vi "MM9.compile header.vi"(0 "i ref in":refnum<vi>, 5 "error in (no error)":errorcluster) -> (14 "i ref out":refnum<vi>, 16 "my header":string, 19 "error out":errorcluster)   [LabVIEW 2014, in "MM9.lvlib"]
doc: "This method compiles the user (Stefan et al.) defined header, that is used in all data files."
uses:
  MM9.lvlib
panel:
  # "This is just for test purposes"
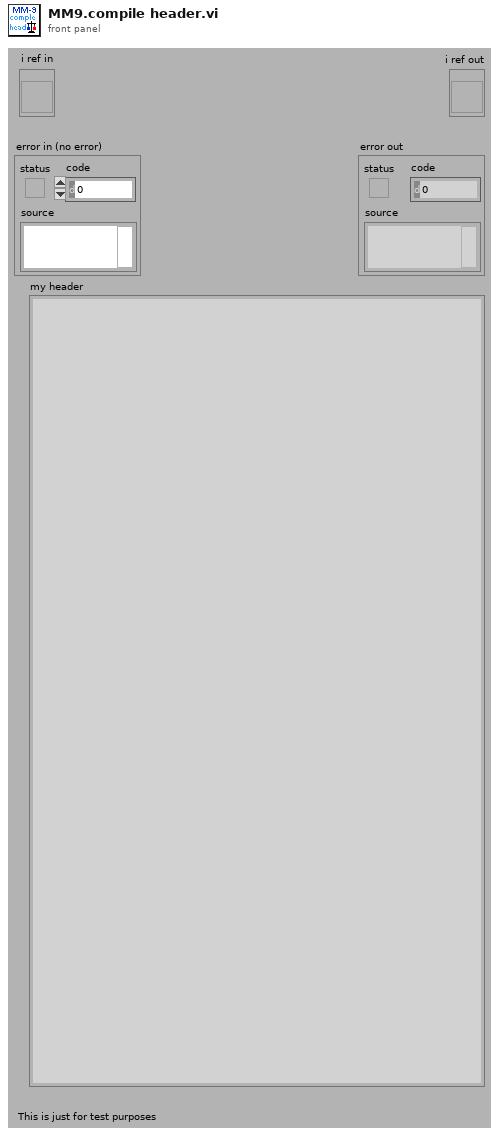
[diagram p1: front panel]
types:
  T1 = typedef "MM9.lvlib/MM9.i attribute.ctl" = cluster{"UsedObjs":string[], "ActScanStep":i32[], "AbortRequest":bool, "StopRequest":bool, "# cycles":i32, "Connected":bool, "MMStatus":T2, "# data":i32, "DIMServices":cluster{"MM6StatusString":string, "MM6StatusID":i32, "discArchiver":string, "discArchiverID":i32, "eventBuilder":string, "eventBuilderID":i32, "GUIIDString":string, "GUIIDStringID":i32}, "dataFile":string, "PGRunning":T3, "ConfigData":T4, "ExtraDataSets":T19}
  T2 = typedef "MM9.lvlib/MM9.status.ctl" = enum16{"loaded", "load_error", "config", "config_error", "init", "init_error", "data_reset", "data_reset_error", "running", "start_error", "run_error", "abort_requested", "aborted", "stop_requested", "stopped", "stop_error", "Connected", "NOTConnected"}
  T3 = typedef "PPG_ABC.lvlib/PPG_ABC.PG_Running.ctl" = i32
  T4 = typedef "LEBITDefs9.lvlib/LEBITDefs.ConfigData.ctl" = cluster{"GenConfig":T5, "Configs":T7[]}
  T5 = typedef "LEBITDefs9.lvlib/LEBITDefs.GenConfig.ctl" = cluster{"Mode":i32, "Logs":T6[]}
  T6 = typedef "LEBITDefs9.lvlib/LEBITDefs.Log.ctl" = cluster{"Name":string, "FctName":string, "Special":string}
  T7 = typedef "LEBITDefs9.lvlib/LEBITDefs.OneConfig.ctl" = cluster{"MCA":T8, "Timing":T9, "Scans":T12[], "FreqDevs":T13[], "CleanDev":T14, "NrCycles":i32, "Specials":T16[], "Delays":T17[], "DAC":T18}
  T8 = typedef "LEBITDefs9.lvlib/LEBITDefs.MCA.ctl" = cluster{"Name":string, "Address":string, "NrChannels":i32, "Gate":i32, "NrPipse":i32, "AcqDelay":i32}
  T9 = typedef "LEBITDefs9.lvlib/LEBITDefs.Timing.ctl" = cluster{"TimeTables":cluster{"TimeTable":T10}[], "Memories":T11[], "ScanX":string, "ScanY":string}
  T10 = typedef "LEBITDefs9.lvlib/LEBITDefs.Timetable.ctl" = dbl[]
  T11 = typedef "LEBITDefs9.lvlib/LEBITDefs.Memory.ctl" = cluster{"Device":string, "ExtTrig":bool, "TT2Use":i32, "PatternTable":string[]}
  T12 = typedef "LEBITDefs9.lvlib/LEBITDefs.ScanDev.ctl" = cluster{"Name":string, "FctName":string, "Values":dbl[], "NrScanVals":i32, "Special":string}
  T13 = typedef "LEBITDefs9.lvlib/LEBITDefs.FreqDev.ctl" = cluster{"Name":string, "Amp":dbl, "CenterFreq":dbl, "Time":dbl}
  T14 = typedef "LEBITDefs9.lvlib/LEBITDefs.CleanDev.ctl" = cluster{"Name":string, "CleanData":T15[]}
  T15 = typedef "LEBITDefs9.lvlib/LEBITDefs.CleanDataType.ctl" = cluster{"Amp":dbl, "Center":dbl, "Plus":dbl, "Minus":dbl, "Time":dbl}
  T16 = typedef "LEBITDefs9.lvlib/LEBITDefs.Special.ctl" = cluster{"Name":string, "FctName":string, "VerySpecial":string, "Data":dbl}
  T17 = typedef "LEBITDefs9.lvlib/LEBITDefs.Delay.ctl" = cluster{"Name":string, "Delay":dbl}
  T18 = typedef "LEBITDefs9.lvlib/LEBITDefs.DAC.ctl" = cluster{"Name":string, "Step1":i32, "Step2":i32}
  T19 = typedef "LEBITDefs9.lvlib/LEBITDefs.ExtraData.ctl" = cluster{"Ions":cluster{"ExcitIonMass":string, "ExcitIonCharge":i32, "CleanIons":cluster{"CleanIonMass":string, "CleanIonCharge":i32}[]}, "TimingDescription":cluster{"TimeTableDescription":cluster{"Times":string[]}[], "PatternTableDescription":cluster{"Pattern":string[]}[]}, "ScanUnits":string[]}[]
  T20 = cluster{"Ions":cluster{"ExcitIonMass":string, "ExcitIonCharge":i32, "CleanIons":cluster{"CleanIonMass":string, "CleanIonCharge":i32}[]}, "TimingDescription":cluster{"TimeTableDescription":cluster{"Times":string[]}[], "PatternTableDescription":cluster{"Pattern":string[]}[]}, "ScanUnits":string[]}
  T21 = cluster{"CleanIonMass":string, "CleanIonCharge":i32}[]
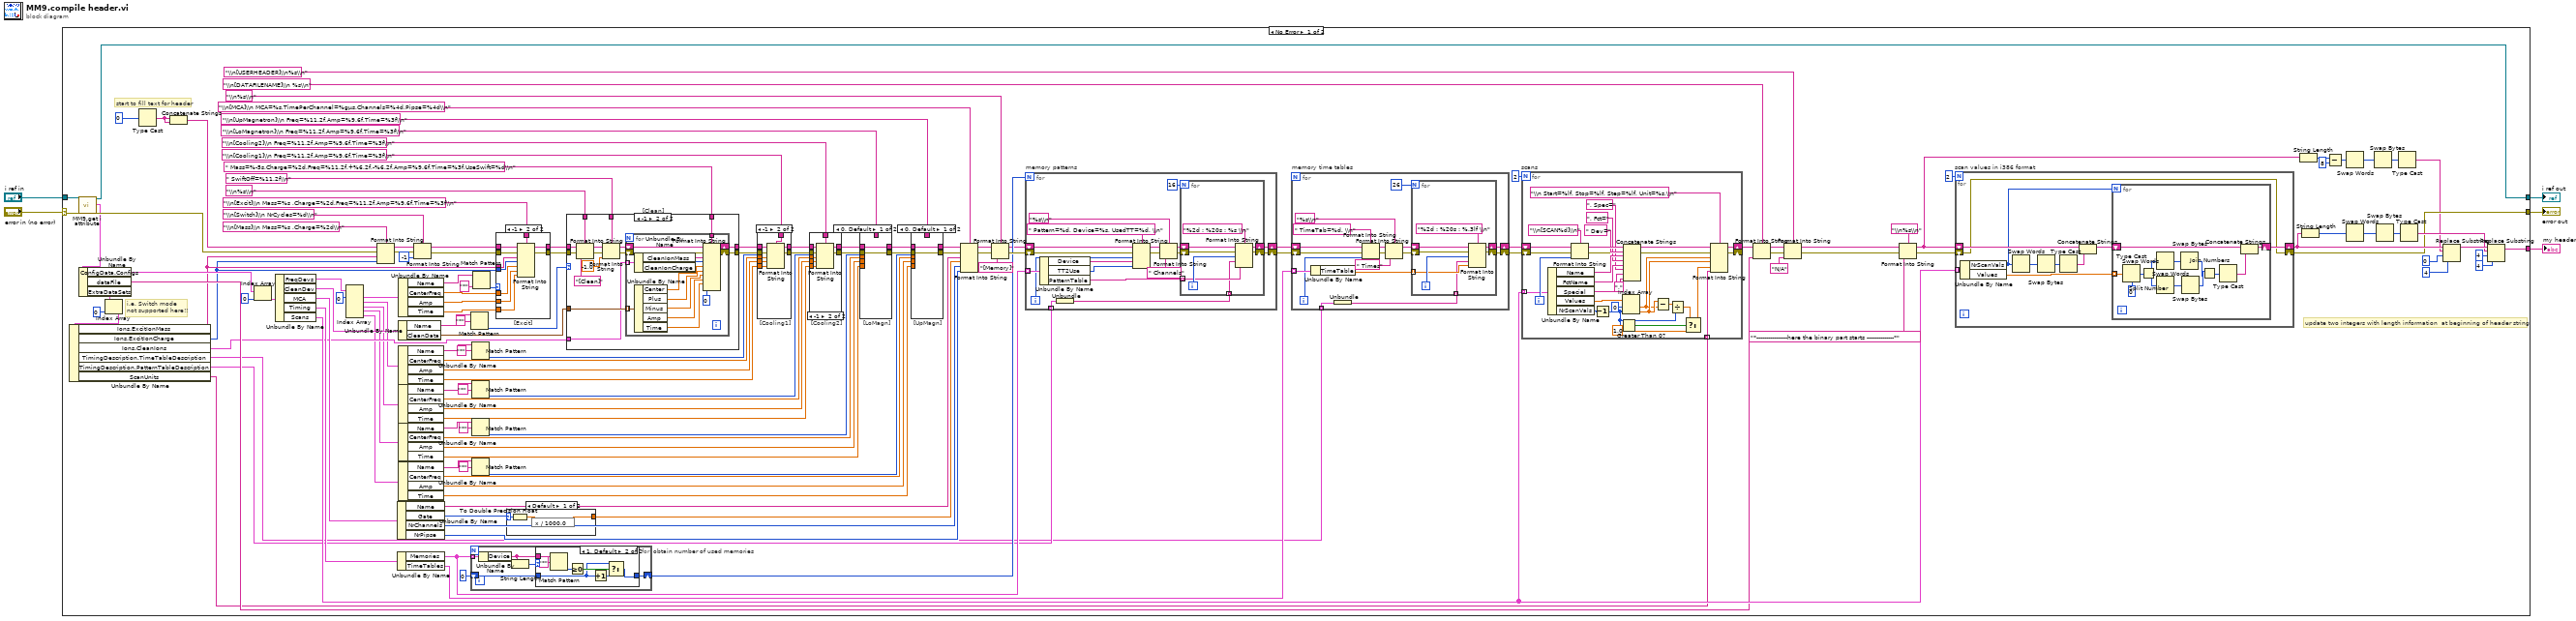
[diagram p0: block diagram]
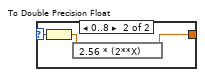
[diagram p3: hidden frame]
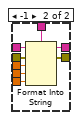
[diagram p4: hidden frame]
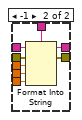
[diagram p5: hidden frame]
diagram:
  n1 = case shown="No Error" "error in (no error)" {
    selector: "error in (no error)" -> [w143 w359]
    tunnel: "i ref in" -> [w147 w360]
    tunnel: [w43 w360] -> w4
    tunnel: [w42 w359] -> w3
    tunnel: [w44 _] -> w1
    frame No Error {
      # "start to fill text for header"
      # "i.e. Switch mode \nnot supported here!!"
      # "update two integers with length information  at beginning of header string"
      n2 = call "MM9.get i attribute.vi"("i ref in"=w147, "error in (no error)"=w143) -> ("i ref out"=w43:refnum<vi>, "i attribute"=w14:T1, "error out"=w137:errorcluster)  [unwired: 15 in]
      n3 = Unbundle By Name(w14) -> ("ConfigData.Configs"=w146:T7[], "dataFile"=w34:string, "ExtraDataSets"=w15:T19)
      n4 = Index Array(array=w15, index=0) -> (element=w20:T20)
      n5 = Unbundle By Name(w20) -> ("Ions.ExcitIonMass"=w19:string, "Ions.ExcitIonCharge"=w18:i32, "Ions.CleanIons"=w13:T21, "TimingDescription.TimeTableDescription"=w16:cluster{"Times":string[]}[], "TimingDescription.PatternTableDescription"=w17:cluster{"Pattern":string[]}[], "ScanUnits"=w12:string[])
      n6 = Type Cast(x=0) -> (*(type *) &x=w149:string)  [unwired: 1 in]
      n7 = Concatenate Strings(w149, w149) -> (w11:string)
      n8 = Index Array(array=w146, index=0) -> (element=w144:T7)
      n9 = Unbundle By Name(w144) -> ("FreqDevs"=w10:T13[], "CleanDev"=w126:T14, "MCA"=w80:T8, "Timing"=w68:T9, "Scans"=w56:T12[])
      n10 = Index Array(array=w10, index #1=0 ("index")) -> (element #1=w133:T13, element #2=w9:T13, element #3=w8:T13, element #4=w7:T13, element #5=w6:T13)  [unwired: 4 in]
      n11 = Format Into String(format string="\\n[Mass]\\n Mass=%s ,Charge=%2d\\n", initial string=w11, error in=w137, w19, w18) -> (resulting string=w141:string, error out=w136:errorcluster)
      n12 = Unbundle By Name(w80) -> ("Name"=w79:string, "Gate"=w78:i32, "NrChannels"=w75:i32, "NrPipse"=w74:i32)
      n13 = Unbundle By Name(w68) -> ("Memories"=w64:T11[], "TimeTables"=w61:cluster{"TimeTable":T10}[])
      n14 = Unbundle By Name(w126) -> ("Name"=w125:string, "CleanData"=w119:T15[])
      n15 = Unbundle By Name(w133) -> ("Name"=w132:string, "CenterFreq"=w129:dbl, "Amp"=w128:dbl, "Time"=w127:dbl)
      n16 = Unbundle By Name(w9) -> ("Name"=w115:string, "CenterFreq"=w110:dbl, "Amp"=w109:dbl, "Time"=w108:dbl)
      n17 = Unbundle By Name(w8) -> ("Name"=w104:string, "CenterFreq"=w101:dbl, "Amp"=w100:dbl, "Time"=w99:dbl)
      n18 = Unbundle By Name(w7) -> ("Name"=w95:string, "CenterFreq"=w93:dbl, "Amp"=w92:dbl, "Time"=w91:dbl)
      n19 = Unbundle By Name(w6) -> ("Name"=w88:string, "CenterFreq"=w86:dbl, "Amp"=w85:dbl, "Time"=w84:dbl)
      n20 = Format Into String(format string="\\n[Switch]\\n NrCycles=%d\\n", initial string=w141, error in=w136, -1 ("input 1")) -> (resulting string=w138:string, error out=w139:errorcluster)
      n21 = for "obtain number of used memories" {
        tunnel: w64 -> [w260] mode=indexing
        shift-right: [w256] -> w66
        shift-left: 0 -> [w257]
        n22 = Unbundle By Name(w260) -> ("Device"=w259:string)
        n23 = String Length(string=w259) -> (length=w258:i32)
        n24 = case shown="1, Default" w258 {
          tunnel: w259 -> [_ w267]
          tunnel: w257 -> [w261 w264]
          tunnel: [w261 w262] -> w256
          frame 0 {
          }
          frame 1, Default {
            n25 = Match Pattern(string=w267, regular expression="*") -> (offset past match=w266:i32)  [unwired: 1 in, 3 out]
            n26 = Greater Or Equal To 0?(x=w266) -> (x >= 0?=w265:bool)
            n27 = Increment(x=w264) -> (x+1=w263:i32)
            n28 = Select(t=w264, s=w265, f=w263) -> (s? t:f=w262:i32)
          }
        }
      }
      n29 = Match Pattern(string=w125, regular expression="*") -> (offset past match=w123:i32)  [unwired: 1 in, 3 out]
      n30 = Match Pattern(string=w115, regular expression="*") -> (offset past match=w112:i32)  [unwired: 1 in, 3 out]
      n31 = Match Pattern(string=w104, regular expression="*") -> (offset past match=w102:i32)  [unwired: 1 in, 3 out]
      n32 = Match Pattern(string=w95, regular expression="*") -> (offset past match=w94:i32)  [unwired: 1 in, 3 out]
      n33 = Match Pattern(string=w88, regular expression="*") -> (offset past match=w87:i32)  [unwired: 1 in, 3 out]
      n34 = Match Pattern(string=w132, regular expression="*") -> (offset past match=w130:i32)  [unwired: 1 in, 3 out]
      n35 = case "[Excit]" shown="-1" w130 {
        tunnel: w139 -> [w347 w358]
        tunnel: w138 -> [w348 w357]
        tunnel: "\\n[Excit]\\n Mass=%s ,Charge=%2d,Freq=%11.2f,Amp=%9.6f,Time=%3f\\n" ("format string") -> [_ w356]
        tunnel: w19 -> [_ w355]
        tunnel: w18 -> [_ w354]
        tunnel: w129 -> [_ w353]
        tunnel: w128 -> [_ w352]
        tunnel: w127 -> [_ w351]
        tunnel: [w348 w350] -> w121
        tunnel: [w347 w349] -> w120
        frame 0, Default {
        }
        frame -1 {
          n36 = Format Into String(format string=w356, initial string=w357, error in=w358, w355, w354, w353, w352, w351) -> (resulting string=w350:string, error out=w349:errorcluster)
        }
      }
      n37 = case shown="Default" w78 {
        selector: w78 -> [w271 w274]
        tunnel: [w270 w273] -> w77
        frame Default {
          n38 = To Double Precision Float(number=w271) -> (double precision float=w269:dbl)
          n39 = expression code="x / 1000.0"(w269) -> (w270:dbl)
        }
        frame 0..8 {
          n40 = To Double Precision Float(number=w274) -> (double precision float=w272:dbl)
          n41 = expression code="2.56 * (2**X)"(w272) -> (w273:dbl)
        }
      }
      n42 = case "[Clean]" shown="-1" w123 {
        tunnel: w120 -> [w315 w328]
        tunnel: w121 -> [w316 w329]
        tunnel: "\\n%s\\n" ("initial string") -> [_ w330]
        tunnel: " SwiftOff=%11.2f\\n" ("initial string") -> [_ w331]
        tunnel: w119 -> [_ w324]
        tunnel: " Mass=%-5s,Charge=%2d,Freq=%11.2f,+%6.2f,-%6.2f,Amp=%9.6f,Time=%3f,UseSwift=%d\\n" ("initial string") -> [_ w321]
        tunnel: [w316 w320] -> w114
        tunnel: [w315 w319] -> w113
        tunnel: w13 -> [_ w317]
        frame 0, Default {
        }
        frame -1 {
          n43 = Format Into String(format string=w330, initial string=w329, error in=w328, "[Clean]") -> (resulting string=w327:string, error out=w325:errorcluster)
          n44 = Format Into String(format string=w331, initial string=w327, error in=w325, -1.0 ("input 1")) -> (resulting string=w323:string, error out=w322:errorcluster)
          n45 = for {
            tunnel: w324 -> [w346] mode=indexing
            tunnel: w321 -> [w345]
            shift-right: [w343] -> w320
            shift-left: w323 -> [w344]
            shift-right: [w342] -> w319
            shift-left: w322 -> [w341]
            tunnel: w317 -> [w337] mode=indexing
            n46 = Unbundle By Name(w337) -> ("CleanIonMass"=w333:string, "CleanIonCharge"=w332:i32)
            n47 = Unbundle By Name(w346) -> ("Center"=w334:dbl, "Plus"=w336:dbl, "Minus"=w335:dbl, "Amp"=w340:dbl, "Time"=w339:dbl)
            n48 = Format Into String(format string=w345, initial string=w344, error in=w341, w333, w332, w334, w336, w335, w340, w339, 0 ("input 8")) -> (resulting string=w343:string, error out=w342:errorcluster)
          }
        }
      }
      n49 = case "[Cooling1]" shown="-1" w112 {
        tunnel: w113 -> [w305 w312]
        tunnel: w114 -> [w306 w313]
        tunnel: "\\n[Cooling1]\\n Freq=%11.2f,Amp=%9.6f,Time=%3f\\n" ("initial string") -> [_ w314]
        tunnel: [w306 w308] -> w106
        tunnel: [w305 w307] -> w107
        tunnel: w110 -> [_ w311]
        tunnel: w109 -> [_ w310]
        tunnel: w108 -> [_ w309]
        frame 0, Default {
        }
        frame -1 {
          n50 = Format Into String(format string=w314, initial string=w313, error in=w312, w311, w310, w309) -> (resulting string=w308:string, error out=w307:errorcluster)
        }
      }
      n51 = case "[Cooling2]" shown="-1" w102 {
        tunnel: w107 -> [w295 w302]
        tunnel: w106 -> [w296 w303]
        tunnel: "\\n[Cooling2]\\n Freq=%11.2f,Amp=%9.6f,Time=%3f\\n" ("initial string") -> [_ w304]
        tunnel: [w296 w298] -> w97
        tunnel: [w295 w297] -> w98
        tunnel: w101 -> [_ w301]
        tunnel: w100 -> [_ w300]
        tunnel: w99 -> [_ w299]
        frame 0, Default {
        }
        frame -1 {
          n52 = Format Into String(format string=w304, initial string=w303, error in=w302, w301, w300, w299) -> (resulting string=w298:string, error out=w297:errorcluster)
        }
      }
      n53 = case "[LoMagn]" shown="0, Default" w94 {
        tunnel: w98 -> [w285 w292]
        tunnel: w97 -> [w286 w293]
        tunnel: "\\n[LoMagnetron]\\n Freq=%11.2f,Amp=%9.6f,Time=%3f\\n" ("initial string") -> [_ w294]
        tunnel: [w286 w288] -> w83
        tunnel: [w285 w287] -> w82
        tunnel: w93 -> [_ w291]
        tunnel: w92 -> [_ w290]
        tunnel: w91 -> [_ w289]
        frame 0, Default {
        }
        frame -1 {
          n54 = Format Into String(format string=w294, initial string=w293, error in=w292, w291, w290, w289) -> (resulting string=w288:string, error out=w287:errorcluster)
        }
      }
      n55 = case "[UpMagn]" shown="0, Default" w87 {
        tunnel: w82 -> [w275 w277]
        tunnel: w83 -> [w276 w283]
        tunnel: "\\n[UpMagnetron]\\n Freq=%11.2f,Amp=%9.6f,Time=%3f\\n" ("initial string") -> [_ w284]
        tunnel: [w276 w279] -> w32
        tunnel: [w275 w278] -> w81
        tunnel: w86 -> [_ w282]
        tunnel: w85 -> [_ w281]
        tunnel: w84 -> [_ w280]
        frame 0, Default {
        }
        frame -1 {
          n56 = Format Into String(format string=w284, initial string=w283, error in=w277, w282, w281, w280) -> (resulting string=w279:string, error out=w278:errorcluster)
        }
      }
      n57 = Format Into String(format string="\\n[MCA]\\n MCA=%s,TimePerChannel=%gµs,Channels=%4d,Pipse=%4d\\n" ("initial string"), initial string=w32, error in=w81, w79, w77, w75, w74) -> (resulting string=w72:string, error out=w71:errorcluster)
      n58 = Format Into String(format string="\\n%s\\n" ("initial string"), initial string=w72, error in=w71, "[Memory]" ("input 1")) -> (resulting string=w65:string, error out=w69:errorcluster)
      n59 = for "memory patterns" {
        N: w66 -> [_]
        shift-right: [w233] -> w63
        shift-left: w65 -> [w246]
        shift-right: [w232] -> w62
        shift-left: w69 -> [w247]
        tunnel: w64 -> [w244] mode=indexing
        tunnel: w17 -> [w230] mode=indexing
        i -> [w243]
        n60 = Unbundle By Name(w244) -> ("Device"=w242:string, "TT2Use"=w241:i32, "PatternTable"=w234:string[])
        n61 = Unbundle(w230) -> ("Pattern"=w229:string[])
        n62 = Format Into String(format string=" Pattern=%d, Device=%s, UsedTT=%d, \\n", initial string=w246, error in=w247, w243, w242, w241) -> (resulting string=w239:string, error out=w240:errorcluster)
        n63 = Format Into String(format string="%s\\n", initial string=w239, error in=w240, " Channels" ("input 1")) -> (resulting string=w237:string, error out=w236:errorcluster)
        n64 = for {
          N: 16 -> [_]
          shift-right: [w251] -> w233
          shift-left: w237 -> [w254]
          tunnel: w234 -> [w252] mode=indexing
          shift-right: [w249] -> w232
          shift-left: w236 -> [w250]
          tunnel: w229 -> [w248] mode=indexing
          i -> [w253]
          n65 = Format Into String(format string="%2d : %20s : %s \\n", initial string=w254, error in=w250, w253, w248, w252) -> (resulting string=w251:string, error out=w249:errorcluster)
        }
      }
      n66 = for "memory time tables" {
        shift-right: [w209] -> w59
        shift-left: w63 -> [w219]
        shift-right: [w208] -> w58
        shift-left: w62 -> [w220]
        tunnel: w61 -> [w217] mode=indexing
        tunnel: w16 -> [w205] mode=indexing
        i -> [w216]
        n67 = Unbundle By Name(w217) -> ("TimeTable"=w207:T10)
        n68 = Unbundle(w205) -> ("Times"=w204:string[])
        n69 = Format Into String(format string=" TimeTab=%d, \\n", initial string=w219, error in=w220, w216) -> (resulting string=w214:string, error out=w215:errorcluster)
        n70 = Format Into String(format string="%s\\n", initial string=w214, error in=w215, " Times" ("input 1")) -> (resulting string=w212:string, error out=w211:errorcluster)
        n71 = for {
          N: 26 -> [_]
          shift-right: [w225] -> w209
          shift-left: w212 -> [w227]
          shift-right: [w223] -> w208
          shift-left: w211 -> [w224]
          tunnel: w207 -> [w222] mode=indexing
          tunnel: w204 -> [w221] mode=indexing
          i -> [w226]
          n72 = Format Into String(format string="%2d : %20s : %.3lf \\n", initial string=w227, error in=w224, w226, w221, w222) -> (resulting string=w225:string, error out=w223:errorcluster)
        }
      }
      n73 = for "scans" {
        N: 2 -> [_]
        shift-right: [w191] -> w36
        shift-left: w59 -> [w182]
        shift-right: [w180] -> _
        shift-left: w58 -> [w203]
        tunnel: w56 -> [w200] mode=indexing
        tunnel: w12 -> [w179] mode=indexing
        i -> [w201]
        n74 = Unbundle By Name(w200) -> ("Name"=w197:string, "FctName"=w195:string, "Special"=w193:string, "Values"=w188:dbl[], "NrScanVals"=w186:i32)
        n75 = Format Into String(format string="\\n[SCAN%d]\\n", initial string=w182, error in=w203, w201) -> (resulting string=w199:string, error out=w181:errorcluster)
        n76 = Decrement(x=w186) -> (x-1=w176:i32)
        n77 = Greater Than 0?(x=w176) -> (x > 0?=w178:bool)
        n78 = Index Array(array=w188, index #1=0 ("index"), index #2=w176) -> (element #1=w184:dbl, element #2=w185:dbl)
        n79 = Concatenate Strings(w199, " Dev=" ("string"), w197, ", Fct=" ("string"), w195, ", Spec=" ("string"), w193, "," ("string")) -> (w190:string)
        n80 = Subtract(x=w185, y=w184) -> (x-y=w183:dbl)
        n81 = Divide(x=w183, y=w176) -> (x/y=w175:dbl)
        n82 = Select(t=w175, s=w178, f=1.0) -> (s? t:f=w174:dbl)
        n83 = Format Into String(format string="\\n Start=%lf, Stop=%lf, Step=%lf, Unit=%s,\\n", initial string=w190, error in=w181, w184, w185, w174, w179) -> (resulting string=w191:string, error out=w180:errorcluster)
      }
      n84 = Format Into String(format string="\\n[DATAFILENAME]\\n %s\\n", initial string=w36, w34) -> (resulting string=w30:string, error out=w29:errorcluster)  [unwired: 1 in]
      n85 = Format Into String(format string="\\n[USERHEADER]\\n%s\\n", initial string=w30, error in=w29, "N/A" ("input 1")) -> (resulting string=w28:string, error out=w27:errorcluster)
      n86 = Format Into String(format string="\\n%s\\n", initial string=w28, error in=w27, "*----------------here the binary part starts --------------*") -> (resulting string=w39:string, error out=w40:errorcluster)
      n87 = for "scan values in i386 format" {
        N: 2 -> [_]
        shift-right: [w153] -> w49
        shift-left: w39 -> [w158]
        shift-right: [w152] -> w42
        shift-left: w40 -> [w152]
        tunnel: w56 -> [w160] mode=indexing
        n88 = Unbundle By Name(w160) -> ("NrScanVals"=w155:i32, "Values"=w151:dbl[])
        n89 = Swap Words(1:w155) -> (0:w159:i32)
        n90 = Swap Bytes(anything=w159) -> (byte swapped=w156:i32)
        n91 = Type Cast(x=w156) -> (*(type *) &x=w157:string)  [unwired: 1 in]
        n92 = Concatenate Strings(w158, w157) -> (w154:string)
        n93 = for {
          N: w155 -> [_]
          shift-right: [w164] -> w153
          shift-left: w154 -> [w163]
          tunnel: w151 -> [w173] mode=indexing
          n94 = Type Cast(type=i64 0, x=w173) -> (*(type *) &x=w171:i64)
          n95 = Split Number(x=w171) -> (hi(x)=w168:u32, lo(x)=w167:u32)
          n96 = Swap Words(1:w168) -> (0:w170:u32)
          n97 = Swap Words(1:w167) -> (0:w169:u32)
          n98 = Swap Bytes(anything=w170) -> (byte swapped=w165:u32)
          n99 = Swap Bytes(anything=w169) -> (byte swapped=w166:u32)
          n100 = Join Numbers(hi=w166, lo=w165) -> ((hi.lo)=w162:u64)
          n101 = Type Cast(x=w162) -> (*(type *) &x=w161:string)  [unwired: 1 in]
          n102 = Concatenate Strings(w163, w161) -> (w164:string)
        }
      }
      n103 = String Length(string=w39) -> (length=w55:i32)
      n104 = String Length(string=w49) -> (length=w24:i32)
      n105 = Subtract(x=w55, y=8) -> (x-y=w22:i32)
      n106 = Swap Words(1:w22) -> (0:w25:i32)
      n107 = Swap Words(1:w24) -> (0:w23:i32)
      n108 = Swap Bytes(anything=w25) -> (byte swapped=w53:i32)
      n109 = Swap Bytes(anything=w23) -> (byte swapped=w52:i32)
      n110 = Type Cast(x=w53) -> (*(type *) &x=w26:string)  [unwired: 1 in]
      n111 = Type Cast(x=w52) -> (*(type *) &x=w47:string)  [unwired: 1 in]
      n112 = Replace Substring(2:4 ("length (len. of substring)"), 3:0 ("offset (0)"), 4:w26, 5:w49) -> (1:w48:string)  [unwired: 1 out]
      n113 = Replace Substring(2:4 ("length (len. of substring)"), 3:4 ("offset (0)"), 4:w47, 5:w48) -> (1:w44:string)  [unwired: 1 out]
    }
    frame Error {
    }
  }
  "error out" <- w3
  "i ref out" <- w4
  "my header" <- w1
